vi "Scalar_Data_4.vi"() -> ()   [LabVIEW 2012]
panel:
  out "Scalar Data 4":u16[](array[numeric])
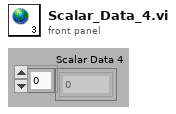
[diagram p1: front panel]
diagram:
